vi "Bertta_v01.vi"() -> ()   [LabVIEW 2015]
uses:
  BERTTA.dll
panel:
  out "Mettler":dynamicdata(graph)
  in  "?":T1(tab)
  out "rc":i32
  in  "Kd":dbl
  in  "Ki":dbl
  in  "Kp":dbl=2.0
  out "PID output":dbl
  in  "Temp setpoint":dbl=20.0
  in  "Device port":dbl=1.0
  out "Debug msg":dbl
  out "Temp Lauda":dbl
  out "Timestep":i32
  in  "Device port":i32=2
  out "Weight":dbl
  out "Weight":dbl
  in  "Device port":i32=6
  out "Lauda":dynamicdata(graph)
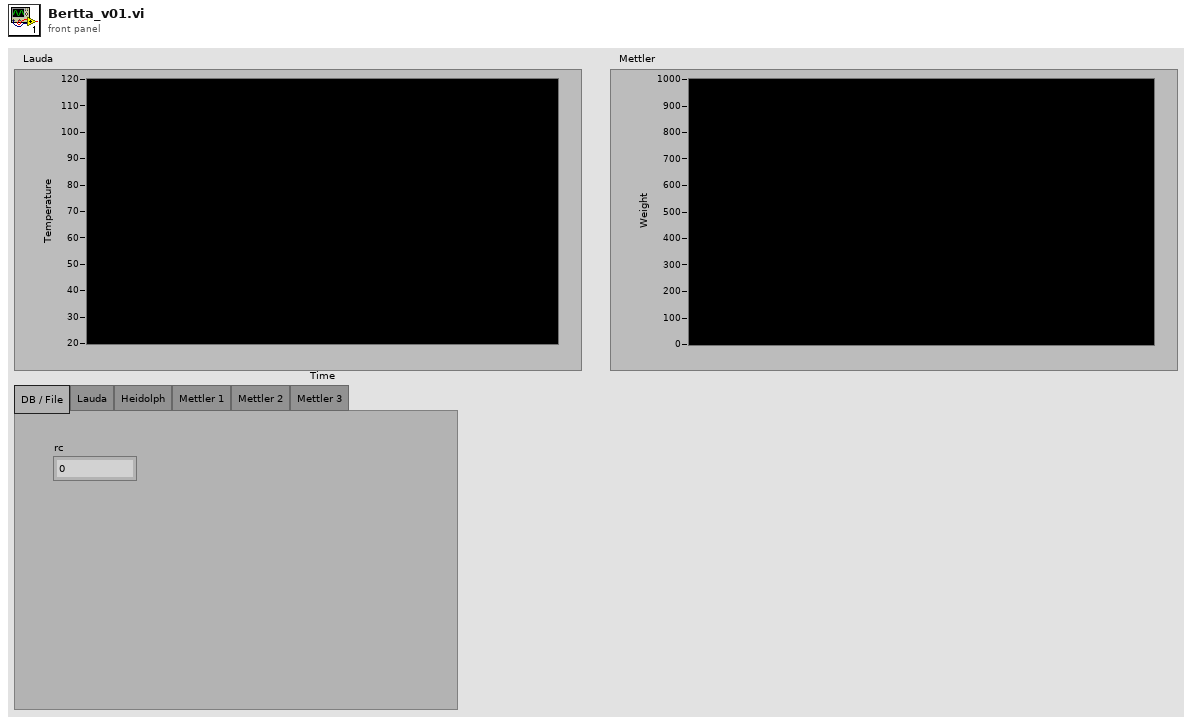
[diagram p1: front panel]
types:
  T1 = enum32{"DB / File", "Lauda", "Heidolph", "Mettler 1", "Mettler 2", "Mettler 3"}
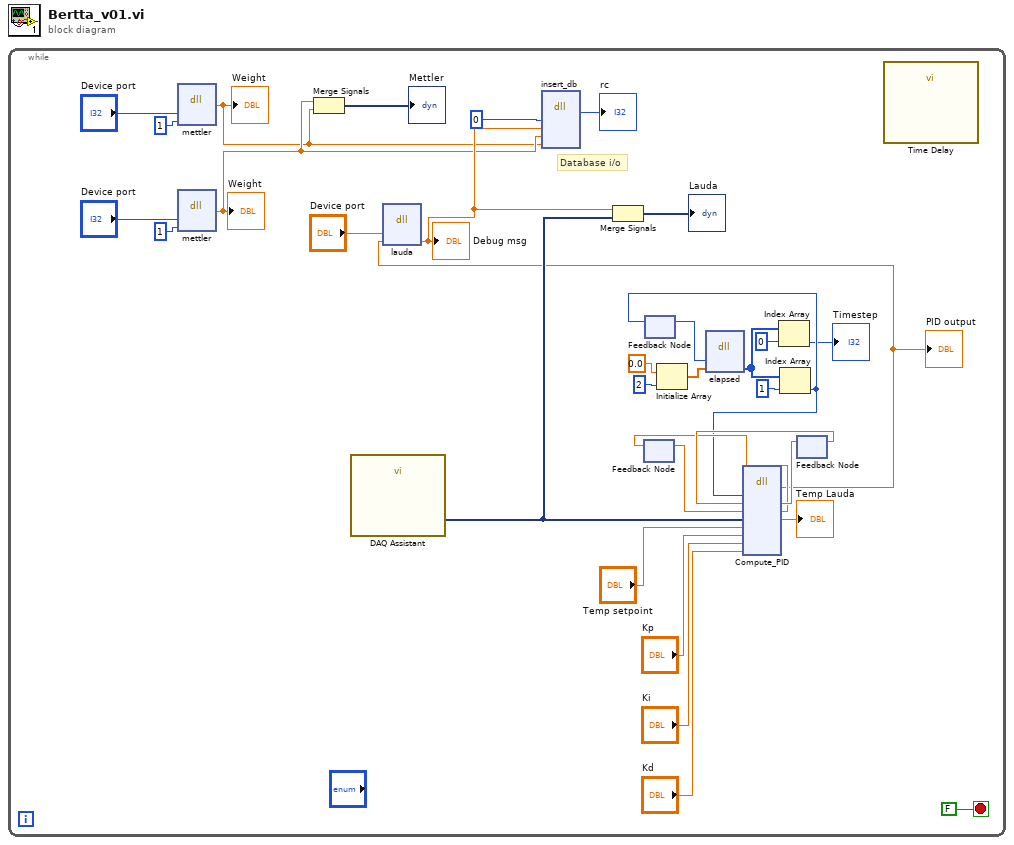
[diagram p0: block diagram]
diagram:
  n1 = while {
    stop <- FALSE stop-if-true
    # "Database i/o"
    n2 = dll-call lib="C:/Users/xlaraser/Documents/Visual Studio 2017/Projects/Bertta/BERTTA/Debug/BERTTA.dll" fn="mettler"("port"="Device port", "msg"=1) -> ("return type"=w11:dbl)  [unwired: 5 in, 2 out]
    "Weight" <- w11
    n3 = dll-call lib="C:/Users/xlaraser/Documents/Visual Studio 2017/Projects/Bertta/BERTTA/Debug/BERTTA.dll" fn="mettler"("port"="Device port", "msg"=1) -> ("return type"=w12:dbl)  [unwired: 5 in, 2 out]
    "Weight" <- w12
    n4 = Merge Signals(w12, w11) -> (→"Mettler":dynamicdata)
    n5 = call "DAQ Assistant"() -> ("data"=w23:dynamicdata)  [unwired: 17 in, 2 out]
    n6 = feedback #1() -> (w27:dbl)  [unwired: 1 in]
    n7 = feedback #2() -> (w8:i32)  [unwired: 1 in]
    n8 = Initialize Array(0.0 ("element"), 2 ("dimension size")) -> (w6:dbl[])
    n9 = dll-call lib="C:/Users/xlaraser/Documents/Visual Studio 2017/Projects/Bertta/BERTTA/Debug/BERTTA.dll" fn="elapsed"("last_time"=w8, "params"=w6) -> ("params"=w2:i32[])  [unwired: 5 in, 2 out]
    n10 = Index Array(array=w2, index=0) -> (element=→"Timestep":i32)
    n11 = Index Array(array=w2, index=1) -> (element=w4:i32)
    n12 = feedback-in #2(w4) -> ()
    n13 = feedback #3() -> (w29:dbl)  [unwired: 1 in]
    n14 = dll-call lib="C:/Users/xlaraser/Documents/Visual Studio 2017/Projects/Bertta/BERTTA/Debug/BERTTA.dll" fn="Compute_PID"("timeChange"=w4, "errSum"=w29, "lastErr"=w27, "Input"=w23, "Setpoint"="Temp setpoint", "kp"="Kp", "ki"="Ki", "kd"="Kd") -> ("return type"=w21:dbl, "errSum"=w30:dbl, "lastErr"=w28:dbl, "Input"=→"Temp Lauda":dbl)  [unwired: 8 in, 2 out]
    "PID output" <- w21
    n15 = dll-call lib="C:/Users/xlaraser/Documents/Visual Studio 2017/Projects/Bertta/BERTTA/Debug/BERTTA.dll" fn="lauda"("port"="Device port", "set_temp"=w21) -> ("set_temp"=w25:dbl)  [unwired: 5 in, 2 out]
    "Debug msg" <- w25
    n16 = dll-call lib="C:/Users/xlaraser/Documents/Visual Studio 2017/Projects/Bertta/BERTTA/Debug/BERTTA.dll" fn="insert_db"("heidolph"=0, "lauda"=w25, "mettler1"=w12, "mettler2"=w11) -> ("return type"=→"rc":i32)  [unwired: 7 in, 2 out]
    n17 = Merge Signals(w25, w23) -> (→"Lauda":dynamicdata)
    n18 = feedback-in #1(w28) -> ()
    n19 = feedback-in #3(w30) -> ()
    n20 = call "Time Delay"() -> ()  [unwired: 11 in, 1 out]
  }
